vi "average_gyro_readings.vi"(2 "Previous gyro readings":i32[](array[numeric]), 3 "Current gyro readings":i32[](array[numeric])) -> (0 "Averaged rotation in YZ":dbl, 1 "Averaged rotation in XZ":dbl)   [LabVIEW 2015]
doc: "Averages the gyro readings from the current and the previous sample taking into acount that readings in XZ plane must be negated in sign. Result is expressed in deg/s"
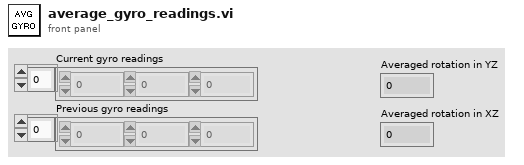
[diagram p1: front panel]
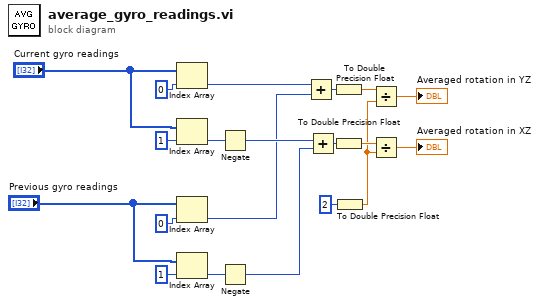
[diagram p0: block diagram]
diagram:
  n1 = Index Array "Index Array"(array="Current gyro readings", index=0) -> (element=w12:i32)
  n2 = Index Array(array="Current gyro readings", index=1) -> (element=w18:i32)
  n3 = Index Array "Index Array"(array="Previous gyro readings", index=0) -> (element=w10:i32)
  n4 = Index Array(array="Previous gyro readings", index=1) -> (element=w16:i32)
  n5 = Negate(x=w18) -> (-x=w11:i32)
  n6 = Negate(x=w16) -> (-x=w9:i32)
  n7 = Add(x=w12, y=w10) -> (x+y=w8:i32)
  n8 = Add(x=w11, y=w9) -> (x+y=w7:i32)
  n9 = To Double Precision Float(number=w8) -> (double precision float=w5:dbl)
  n10 = To Double Precision Float(number=w7) -> (double precision float=w4:dbl)
  n11 = To Double Precision Float(number=2 ("y")) -> (double precision float=w3:dbl)
  n12 = Divide(x=w5, y=w3) -> (x/y=→"Averaged rotation in YZ":dbl)
  n13 = Divide(x=w4, y=w3) -> (x/y=→"Averaged rotation in XZ":dbl)
